vi "Position Tracking.vi"() -> ()   [LabVIEW 2019]
uses:
  Position Data.vi
  Globals/Sensor_Values.vi
  <vilib>/Utility/file.llb/Read Delimited Spreadsheet (DBL).vi
panel:
  in  "Rotations to distance(ft) multiplier":dbl
  out "X and Y pos":cluster{dbl, dbl}(graph)
  out "Pigeon Yaw":cluster{"Yaw":dbl}(graph)
  out "XY Graph":cluster{"array":dbl[], "array":dbl[]}[](graph)
  out "Y position":dbl
  out "X position":dbl
  out "Dist from origin":dbl
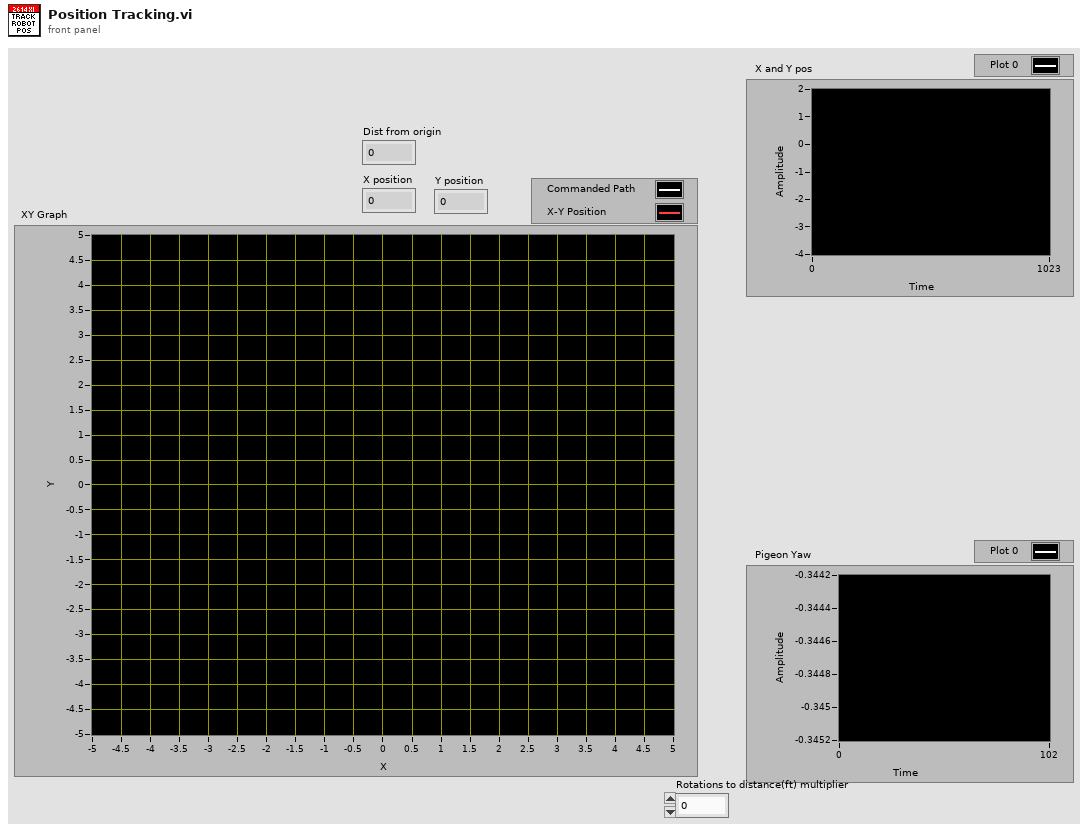
[diagram p1: front panel]
types:
  T1 = typedef "CTRE_PigeonIMU_DeviceRef.ctl" = cluster{"DeviceStatus":errorcluster, "Device Number":u8, "Type":T2, "Device ID":u32, "Handle":u64, "UsageFrame":u32, "Library Path":path}
  T2 = typedef "CTRE_PigeonIMU_ConnectionType.ctl" = u32
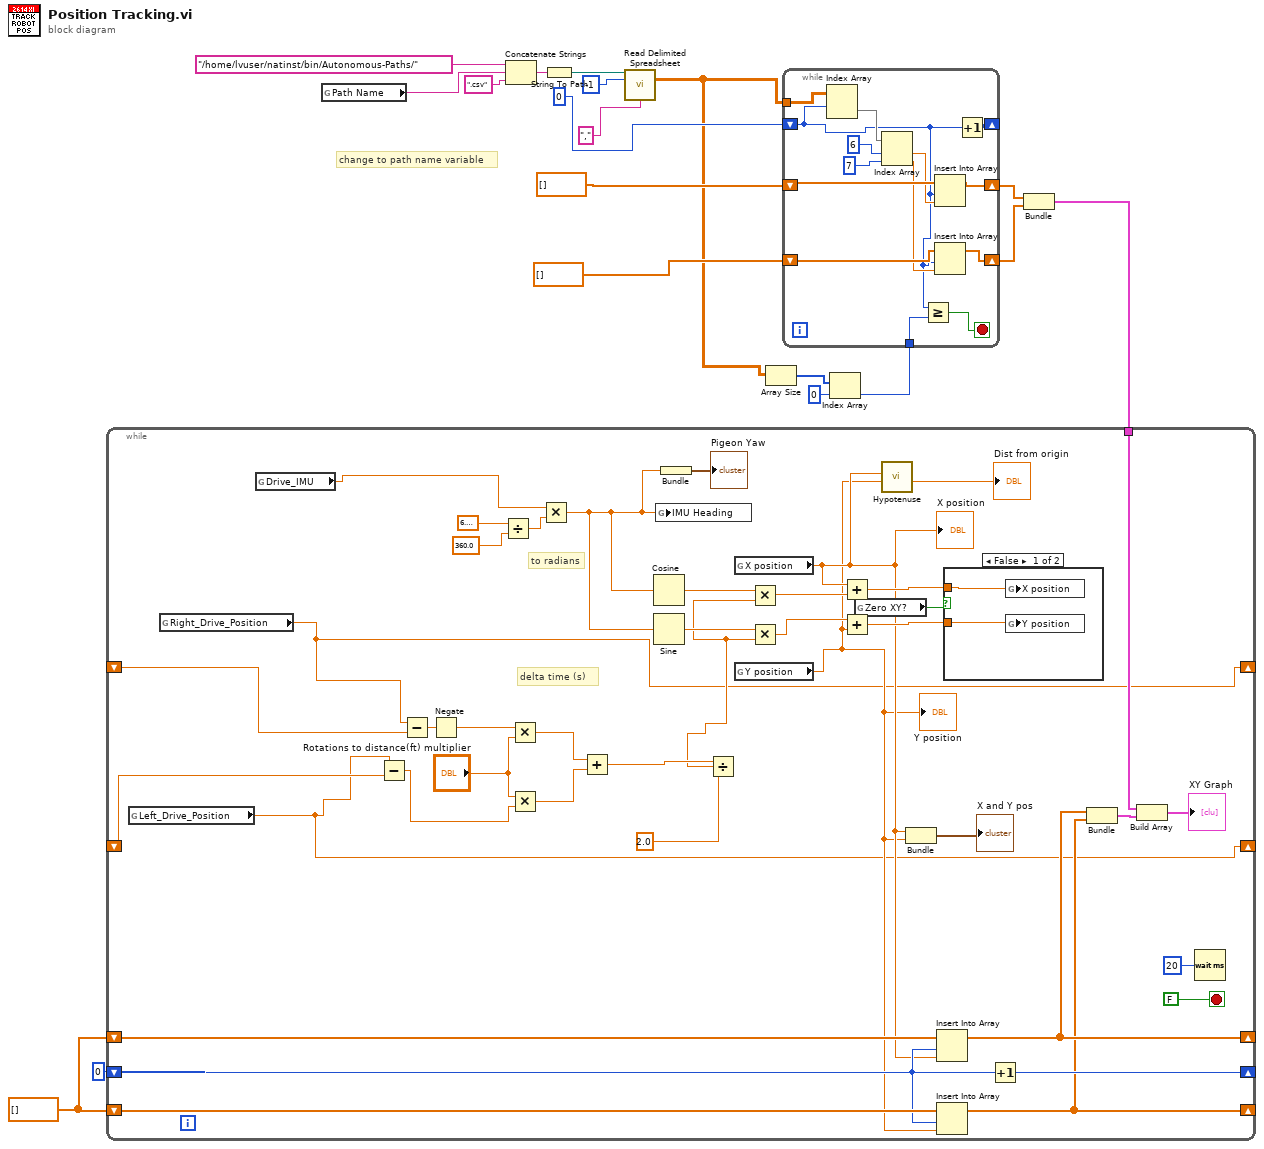
[diagram p0: block diagram]
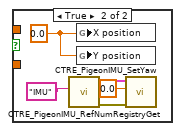
[diagram p2: hidden frame]
diagram:
  w18 = dbl[] [] ("array")
  # "change to path name variable"
  n1 = global read "Position Data.vi" "Path Name"() -> (w1:string)
  n2 = Concatenate Strings("/home/lvuser/natinst/bin/Autonomous-Paths/", w1, ".csv" ("string")) -> (w14:string)
  n3 = String To Path(string=w14) -> (path=w13:path)
  n4 = call-poly <vilib>:"Read Delimited Spreadsheet.vi"("file path (dialog if empty)"=w13, "number of rows (all:-1)"=-1, "delimiter (\\t)"="," ("delimiter (\\t)")) -> ("all rows"=w8:dbl[][])  [unwired: 7 in, 5 out]
  n5 = Array Size(array=w8) -> (size(s)=w7:i32[])
  n6 = Index Array(array=w7, index=0) -> (element=w5:i32)
  n7 = while {
    tunnel: w8 -> [w33]
    shift-right: [w32] -> _
    shift-left: 0 ("index (row)") -> [w23]
    shift-right: [w21] -> w4
    shift-left: dbl[] [] ("array") -> [w28]
    shift-right: [w20] -> w3
    shift-left: dbl[] [] ("array") -> [w27]
    tunnel: w5 -> [w24]
    stop <- w22 stop-if-true
    n8 = Index Array(array=w33, index (row)=w23) -> (element=w31:dbl[])  [unwired: 1 in]
    n9 = Index Array(array=w31, index #1=6 ("index"), index #2=7 ("index")) -> (element #1=w26:dbl, element #2=w25:dbl)
    n10 = Greater Or Equal?(x=w23, y=w24) -> (x >= y?=w22:bool)
    n11 = Insert Into Array(array=w28, index=w23, new element=w26) -> (w21:dbl[])
    n12 = Insert Into Array(array=w27, index=w23, new element=w25) -> (w20:dbl[])
    n13 = Increment(x=w23) -> (x+1=w32:i32)
  }
  n14 = Bundle("array"=w4, "array"=w3) -> (w2:cluster{"array":dbl[], "array":dbl[]})  [unwired: 1 in]
  n15 = while {
    shift-right: [w60] -> _
    shift-left: w18 -> [w64]
    shift-right: [w59] -> _
    shift-left: w18 -> [w63]
    shift-right: [w62] -> _
    shift-left: 0 ("index") -> [w61]
    tunnel: w2 -> [w56]
    shift-right: [w37] -> _
    shift-left: _ -> [w36]
    shift-right: [w34] -> _
    shift-left: _ -> [w35]
    stop <- FALSE stop-if-true
    # "to radians"
    # "delta time (s)"
    n16 = global read "Sensor_Values.vi" "Left_Drive_Position"() -> (w34:dbl)
    n17 = global read "Sensor_Values.vi" "Right_Drive_Position"() -> (w37:dbl)
    n18 = global read "Sensor_Values.vi" "Drive_IMU"() -> (w39:dbl)
    n19 = Subtract(x=w34, y=w35) -> (x-y=w47:dbl)
    n20 = Subtract(x=w37, y=w36) -> (x-y=w52:dbl)
    n21 = Negate(x=w52) -> (-x=w46:dbl)
    n22 = Divide(x=6.283185307179586, y=360.0) -> (x/y=w53:dbl)
    n23 = Multiply(x=w46, y="Rotations to distance(ft) multiplier") -> (x*y=w49:dbl)
    n24 = Multiply(x="Rotations to distance(ft) multiplier", y=w47) -> (x*y=w48:dbl)
    n25 = Multiply(x=w39, y=w53) -> (x*y=w44:dbl)
    n26 = Add(x=w49, y=w48) -> (x+y=w51:dbl)
    n27 = Cosine(x=w44) -> (cos(x)=w72:dbl)
    n28 = Sine(x=w44) -> (sin(x)=w70:dbl)
    n29 = global write "Position Data.vi" "IMU Heading"(w44) -> ()
    n30 = Bundle(w44) -> (→"Pigeon Yaw":cluster{dbl})  [unwired: 1 in]
    n31 = Divide(x=w51, y=2.0) -> (x/y=w40:dbl)
    n32 = global read "Position Data.vi" "X position"() -> (w43:dbl)
    "X position" <- w43
    n33 = global read "Position Data.vi" "Y position"() -> (w42:dbl)
    "Y position" <- w42
    n34 = Multiply(x=w72, y=w40) -> (x*y=w71:dbl)
    n35 = Multiply(x=w70, y=w40) -> (x*y=w69:dbl)
    n36 = Add(x=w43, y=w71) -> (x+y=w67:dbl)
    n37 = Add(x=w69, y=w42) -> (x+y=w66:dbl)
    n38 = global read "Position Data.vi" "Zero XY?"() -> (w45:bool)
    n39 = call "Hypotenuse.vi"("b"=w42, "a"=w43) -> ("c"=→"Dist from origin":dbl)  [unwired: 9 in]
    n40 = Bundle("X position"=w43, "Y position"=w42) -> (→"X and Y pos":cluster{"X position":dbl, "Y position":dbl})  [unwired: 1 in]
    n41 = Insert Into Array(array=w64, index=w61, new element=w43) -> (w60:dbl[])
    n42 = Insert Into Array(array=w63, index=w61, new element=w42) -> (w59:dbl[])
    n43 = case shown="False" w45 {
      tunnel: w67 -> [w76 _]
      tunnel: w66 -> [w75 _]
      frame False {
        n44 = global write "Position Data.vi" "X position"(w76) -> ()
        n45 = global write "Position Data.vi" "Y position"(w75) -> ()
      }
      frame True {
        w81 = 0.0 ("X position")
        n46 = call <vilib>:"CTRE_PigeonIMU_RefNumRegistryGet.vi"("refnum name"="IMU") -> ("error out"=w78:errorcluster, "PigeonIMUDevRef"=w77:T1)  [unwired: 9 in]
        n47 = global write "Position Data.vi" "X position"(w81) -> ()
        n48 = global write "Position Data.vi" "Y position"(w81) -> ()
        n49 = call <vilib>:"CTRE_PigeonIMU_SetYaw.vi"("error in (no error)"=w78, "Value"=0.0, "PigeonIMUDevRef"=w77) -> ()  [unwired: 7 in, 2 out]
      }
    }
    n50 = Increment(x=w61) -> (x+1=w62:i32)
    n51 = Bundle("array"=w60, "array"=w59) -> (w58:cluster{"array":dbl[], "array":dbl[]})  [unwired: 1 in]
    n52 = Build Array(w56, w58) -> (→"XY Graph":cluster{"array":dbl[], "array":dbl[]}[])
    n53 = Wait (ms)(milliseconds to wait=u32 20) -> ()  [unwired: 1 out]
  }
